vi "ManageUSB.vi"(8 "error in (no error)":errorcluster, 10 "USB root":path, 11 "Qbus in":refnum<class "Qbus.lvclass">) -> (0 "error out":errorcluster)   [LabVIEW 2017, in "USBDrive.lvlib"]
uses:
  <vilib>/addons/InsightCM/Devices/Shared/Common/USBDrive/USBDrive.lvlib
  <vilib>/addons/Qbus/Qbus.lvclass
  <vilib>/addons/BlinkProcess/controls/mode.ctl
  <vilib>/addons/BlinkProcess/BlinkProcess.lvlib
  <vilib>/addons/SystemInfoProcess/SystemInfoProcess.lvlib
  <vilib>/addons/InsightCM/Devices/Shared/Common/ServerComm/ServerComm.lvlib
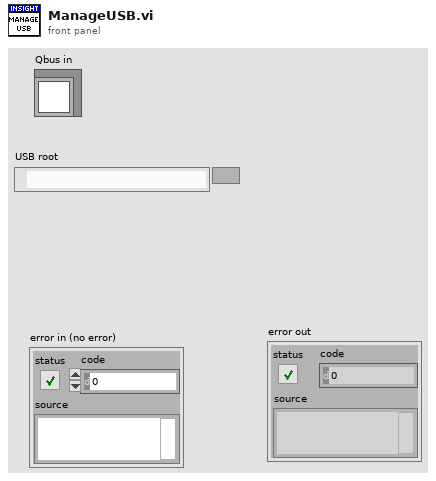
[diagram p1: front panel]
types:
  T1 = typedef "BlinkProcess.lvlib/mode.ctl" = enum16{"Normal", "Error", "On", "Off", "Custom"}
  T2 = typedef "ConnectionInfo.ctl" = cluster{"ClientName":string, "TransceiverHost":string, "TransceiverPort":u16, "Password":string}
  T3 = typedef "SystemInfoProcess.lvlib/NetworkAdapterSettings.ctl" = cluster{"Adapter Mode":u32, "IsPrimary":bool, "MACAddr":string, "IP Address Request Mode":u32, "IPAddr":string, "SubnetMask":string, "Gateway":string, "DNSServer":string, "Alias":string}
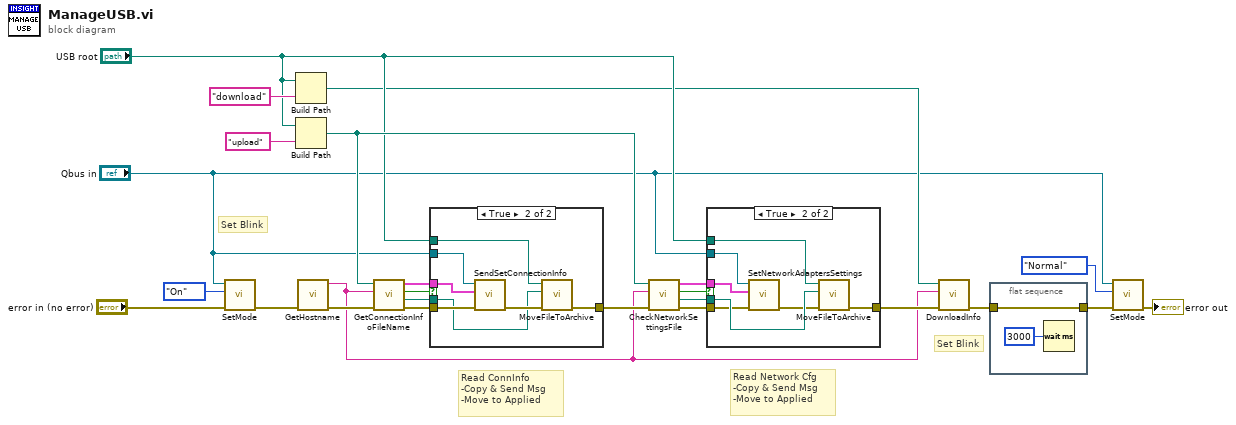
[diagram p0: block diagram]
diagram:
  # "Read Network Cfg\n-Copy & Send Msg\n-Move to Applied"
  # "Read ConnInfo\n-Copy & Send Msg\n-Move to Applied"
  # "Set Blink"
  # "Set Blink"
  n1 = call <vilib>:"SetMode.vi"("error in (no error)"="error in (no error)", "mode"=mode."On", "Qbus in"="Qbus in") -> ("error out"=w23:errorcluster)  [unwired: 7 in, 1 out]
  n2 = Build Path(base path="USB root", name or relative path="download") -> (appended path=w8:path)
  n3 = Build Path(base path="USB root", name or relative path="upload") -> (appended path=w15:path)
  n4 = call <vilib>:"GetHostname.vi"("error in (no error)"=w23) -> ("error out"=w22:errorcluster, "hostname"=w7:string)  [unwired: 9 in]
  n5 = call <vilib>:"GetConnectionInfoFileName.vi"("error in (no error)"=w22, "hostname"=w7, "upload path"=w15) -> ("error out"=w21:errorcluster, "connInfo file"=w16:path, "exists"=w17:bool, "connection info"=w20:T2)  [unwired: 5 in]
  n6 = case shown="True" w17 {
    tunnel: w21 -> [w26 w33]
    tunnel: w20 -> [_ w31]
    tunnel: "Qbus in" -> [_ w32]
    tunnel: "USB root" -> [_ w29]
    tunnel: [w26 w28] -> w18
    tunnel: w16 -> [_ w27]
    frame False {
    }
    frame True {
      n7 = call <vilib>:"SendSetConnectionInfo.vi"("error in (no error)"=w33, "connection info"=w31, "Qbus in"=w32) -> ("error out"=w30:errorcluster)  [unwired: 7 in, 1 out]
      n8 = call <vilib>:"MoveFileToArchive.vi"("error in (no error)"=w30, "Source File"=w27, "USB root"=w29) -> ("error out"=w28:errorcluster)  [unwired: 8 in]
    }
  }
  n9 = call <vilib>:"CheckNetworkSettingsFile.vi"("error in (no error)"=w18, "hostname"=w7, "upload path"=w15) -> ("error out"=w14:errorcluster, "path"=w11:path, "exists"=w13:bool, "NetworkSettings"=w12:T3[])  [unwired: 5 in]
  n10 = case shown="True" w13 {
    tunnel: w14 -> [w34 w38]
    tunnel: w12 -> [_ w35]
    tunnel: "Qbus in" -> [_ w36]
    tunnel: "USB root" -> [_ w41]
    tunnel: [w34 w40] -> w9
    tunnel: w11 -> [_ w39]
    frame False {
    }
    frame True {
      n11 = call <vilib>:"SetNetworkAdaptersSettings.vi"("error in (no error)"=w38, "NetworkSettings"=w35, "Qbus in"=w36) -> ("error out"=w37:errorcluster)  [unwired: 8 in]
      n12 = call <vilib>:"MoveFileToArchive.vi"("error in (no error)"=w37, "Source File"=w39, "USB root"=w41) -> ("error out"=w40:errorcluster)  [unwired: 8 in]
    }
  }
  n13 = call <vilib>:"DownloadInfo.vi"("error in (no error)"=w9, "hostname"=w7, "USB download"=w8) -> ("error out"=w5:errorcluster)  [unwired: 8 in]
  n14 = flat-sequence {
    tunnel: [w43] -> w6
    tunnel: w5 -> [w43]
    frame #0 {
      n15 = Wait (ms)(milliseconds to wait=u32 3000) -> ()  [unwired: 1 out]
    }
  }
  n16 = call <vilib>:"SetMode.vi"("error in (no error)"=w6, "mode"=mode."Normal", "Qbus in"="Qbus in") -> ("error out"=→"error out":errorcluster)  [unwired: 7 in, 1 out]
